vi "ResistanceProtocol.vi"() -> (1 "ResistanceProtocol":string, 2 "output 1":i32, 3 "outputProtocol":string)   [LabVIEW 2018]
uses:
  Global Variables.vi
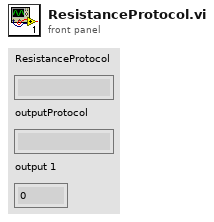
[diagram p1: front panel]
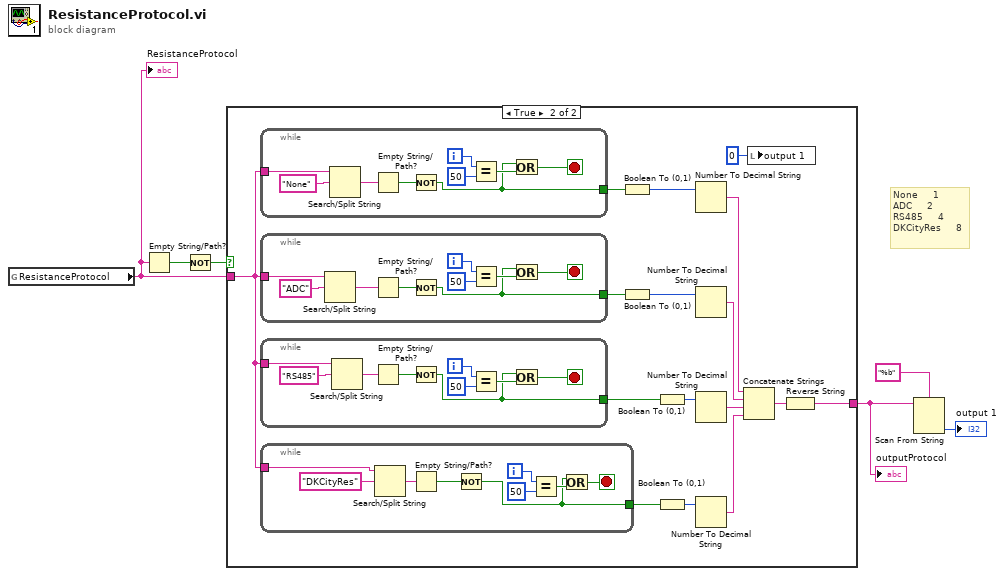
[diagram p0: block diagram]
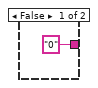
[diagram p2: hidden frame]
diagram:
  # "None     1\nADC     2\nRS485     4\nDKCityRes     8"
  n1 = global read "Global Variables.vi" "ResistanceProtocol"() -> (w1:string)
  "ResistanceProtocol" <- w1
  n2 = Empty String/Path?(string/path=w1) -> (empty?=w3:bool)
  n3 = Not(x=w3) -> (.not. x?=w2:bool)
  n4 = case shown="True" w2 {
    tunnel: w1 -> [_ w10]
    tunnel: ["0" w9] -> w5
    frame False {
    }
    frame True {
      n5 = while {
        tunnel: [w52] -> w22
        tunnel: w10 -> [w51]
        i -> [w59]
        stop <- w57 stop-if-true
        n6 = Search/Split String(string=w51, search string/char (-)="None") -> (match + rest of string=w53:string)  [unwired: 1 in, 2 out]
        n7 = Empty String/Path?(string/path=w53) -> (empty?=w54:bool)
        n8 = Not(x=w54) -> (.not. x?=w52:bool)
        n9 = Equal?(x=w59, y=50) -> (x = y?=w56:bool)
        n10 = Or(x=w52, y=w56) -> (x .or. y?=w57:bool)
      }
      n11 = while {
        tunnel: [w43] -> w18
        tunnel: w10 -> [w42]
        i -> [w50]
        stop <- w48 stop-if-true
        n12 = Search/Split String(string=w42, search string/char (-)="ADC") -> (match + rest of string=w44:string)  [unwired: 1 in, 2 out]
        n13 = Empty String/Path?(string/path=w44) -> (empty?=w45:bool)
        n14 = Not(x=w45) -> (.not. x?=w43:bool)
        n15 = Equal?(x=w50, y=50) -> (x = y?=w47:bool)
        n16 = Or(x=w43, y=w47) -> (x .or. y?=w48:bool)
      }
      n17 = while {
        tunnel: [w34] -> w17
        tunnel: w10 -> [w33]
        i -> [w41]
        stop <- w39 stop-if-true
        n18 = Search/Split String(string=w33, search string/char (-)="RS485") -> (match + rest of string=w35:string)  [unwired: 1 in, 2 out]
        n19 = Empty String/Path?(string/path=w35) -> (empty?=w36:bool)
        n20 = Not(x=w36) -> (.not. x?=w34:bool)
        n21 = Equal?(x=w41, y=50) -> (x = y?=w38:bool)
        n22 = Or(x=w34, y=w38) -> (x .or. y?=w39:bool)
      }
      n23 = while {
        tunnel: [w25] -> w16
        tunnel: w10 -> [w24]
        i -> [w32]
        stop <- w30 stop-if-true
        n24 = Search/Split String(string=w24, search string/char (-)="DKCityRes") -> (match + rest of string=w26:string)  [unwired: 1 in, 2 out]
        n25 = Empty String/Path?(string/path=w26) -> (empty?=w27:bool)
        n26 = Not(x=w27) -> (.not. x?=w25:bool)
        n27 = Equal?(x=w32, y=50) -> (x = y?=w29:bool)
        n28 = Or(x=w25, y=w29) -> (x .or. y?=w30:bool)
      }
      n29 = Boolean To (0,1)(Boolean=w22) -> (0, 1=w23:i16)
      n30 = Boolean To (0,1)(Boolean=w18) -> (0, 1=w21:i16)
      n31 = Boolean To (0,1)(Boolean=w17) -> (0, 1=w20:i16)
      n32 = Boolean To (0,1)(Boolean=w16) -> (0, 1=w19:i16)
      n33 = Number To Decimal String(number=w23) -> (decimal integer string=w15:string)  [unwired: 1 in]
      n34 = Number To Decimal String(number=w21) -> (decimal integer string=w14:string)  [unwired: 1 in]
      n35 = Number To Decimal String(number=w20) -> (decimal integer string=w13:string)  [unwired: 1 in]
      n36 = Number To Decimal String(number=w19) -> (decimal integer string=w12:string)  [unwired: 1 in]
      n37 = Concatenate Strings(w15, w14, w13, w12) -> (w11:string)
      n38 = local write "output 1"(0 ("output 1")) -> ()
      n39 = Reverse String(1:w11) -> (0:w9:string)
    }
  }
  "outputProtocol" <- w5
  n40 = Scan From String(format string="%b", input string=w5) -> (output 1=→"output 1":i32)  [unwired: 3 in, 3 out]
